vi "PreOrderTraverse1.vi"(6 "error in (no error)":errorcluster caption="错误输入（无错误）", 7 "Data in":variant, 8 "Method Name":string, 9 "Node* in":refnum<data-value>) -> (0 "error out":errorcluster caption="错误输出", 1 "Data out":variant, 3 "Node* out":refnum<data-value>)   [LabVIEW 2013, in "PanelLinkNode.lvclass"]
uses:
  PanelLinkNode.lvclass
  PanelLinkNode.lvclass/PanelLinkNode.ctl
  PanelObject/PanelObject.lvclass
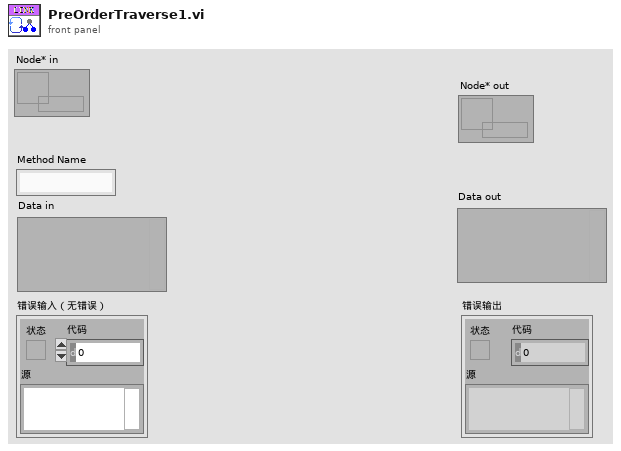
[diagram p1: front panel]
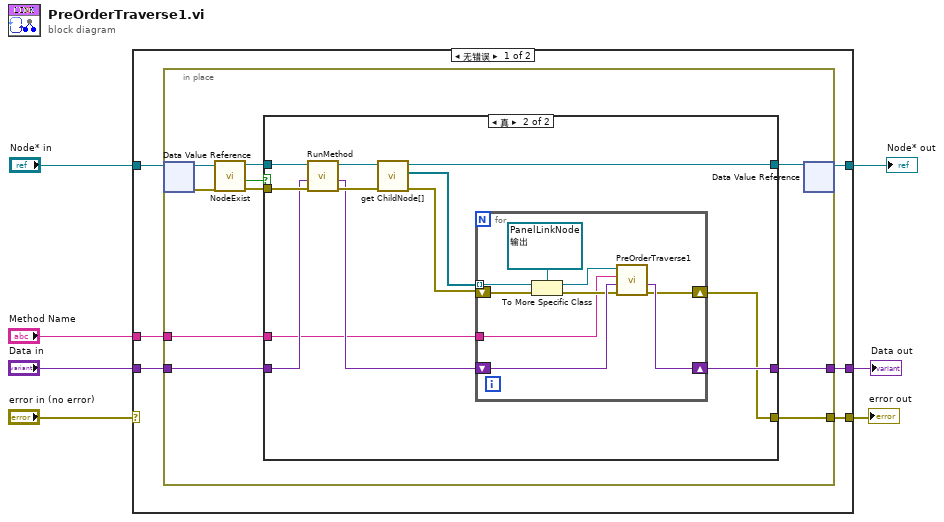
[diagram p0: block diagram]
diagram:
  n1 = case shown="无错误" "error in (no error)" {
    selector: "error in (no error)" -> [_ w50]
    tunnel: [w9 w50] -> w6
    tunnel: "Node* in" -> [w13 w48]
    tunnel: "Method Name" -> [w12 _]
    tunnel: "Data in" -> [w11 w49]
    tunnel: [w10 w49] -> w2
    tunnel: [w8 w48] -> w1
    frame No Error {
      n2 = in-place {
        in-place-border: w12 -> [w18]
        in-place-border: w11 -> [w17]
        in-place-border: [w16] -> w10
        in-place-border: [w14] -> w9
        n3 = in-place-dvr #1(w13) -> (w23:refnum<class "PanelLinkNode.lvclass">, w22:errorcluster)
        n4 = call-dynamic "NodeExist.vi"("error in (no error)"=w22, "PanelLinkNode 输入"=w23) -> ("error out"=w19:errorcluster, "Node Exist?"=w21:bool, "PanelLinkNode 输出"=w20:refnum<class "PanelLinkNode.lvclass">)  [unwired: 7 in]
        n5 = case shown="真" w21 {
          tunnel: w20 -> [w25 w38]
          tunnel: w19 -> [w24 w37]
          tunnel: w18 -> [_ w27]
          tunnel: w17 -> [w26 w36]
          tunnel: [w26 w31] -> w16
          tunnel: [w25 w29] -> w15
          tunnel: [w24 w28] -> w14
          frame False {
          }
          frame True {
            n6 = call-dynamic "RunMethod.vi"("error in (no error)"=w37, "Data in"=w36, "PanelLinkNode 输入"=w38) -> ("error out"=w34:errorcluster, "Data out"=w32:variant, "PanelLinkNode 输出"=w35:refnum<class "PanelLinkNode.lvclass">)  [unwired: 4 in, 2 out]
            n7 = call "get ChildNode[].vi"("error in (no error)"=w34, "PanelLinkNode输入"=w35) -> ("error out"=w30:errorcluster, "ChildNode*[]"=w33:refnum<data-value>[], "PanelLinkNode输出"=w29:refnum<class "PanelLinkNode.lvclass">)  [unwired: 7 in]
            n8 = for {
              tunnel: w33 -> [w46] mode=indexing
              shift-right: [w44] -> w31
              shift-left: w32 -> [w45]
              shift-right: [w41] -> w28
              shift-left: w30 -> [w43]
              tunnel: w27 -> [w39]
              n9 = To More Specific Class(target class=refnum<data-value> refnum ("数据值引用"), reference=w46, error in=w43) -> (specific class reference=w40:refnum<data-value>, error out=w42:errorcluster)
              n10 = call "PreOrderTraverse1.vi"("error in (no error)"=w42, "Data in"=w45, "Method Name"=w39, "Node* in"=w40) -> ("error out"=w41:errorcluster, "Data out"=w44:variant)  [unwired: 3 in, 1 out]
            }
          }
        }
        n11 = in-place-dvr #1(w15) -> (w8:refnum<data-value>)  [unwired: 1 out]
      }
    }
    frame Error {
    }
  }
  "error out" <- w6
  "Data out" <- w2
  "Node* out" <- w1
